vi "Get Language Name.vi"(8 "error in (no error)":errorcluster) -> (0 "error out":errorcluster, 1 "Path":map{string, path}(c390), 2 "Tag":string[](array[string]), 3 "Tag Name":string[](array[string]))   [LabVIEW 2025, in "Localization.lvlib"]
uses:
  Localization.lvlib
  <vilib>/Utility/config.llb/Read Key (String).vi
  Full User Interface/Full User Interface.lvlib
  <userlib>/_OpenG.lib/file/file.llb/openg_file.lvlib
  <vilib>/Utility/config.llb/NI_LVConfig.lvlib
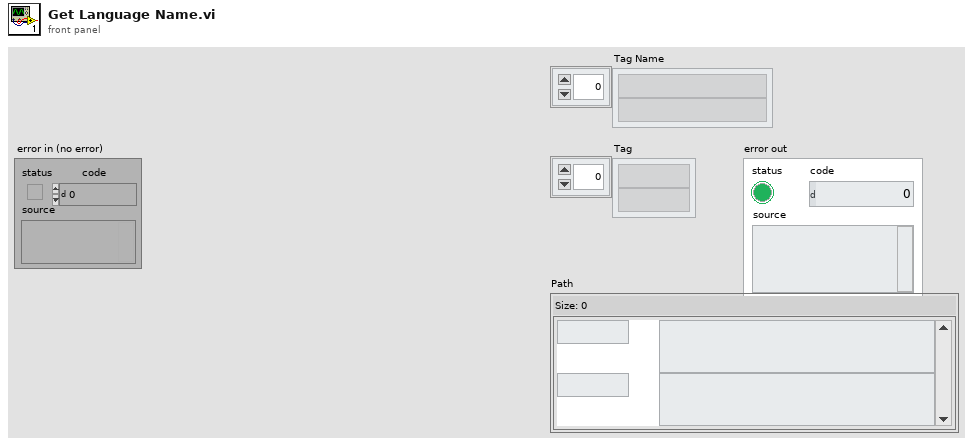
[diagram p1: front panel]
types:
  T1 = typedef "NI_LVConfig.lvlib/Config Data RefNum.ctl" = refnum<k1>
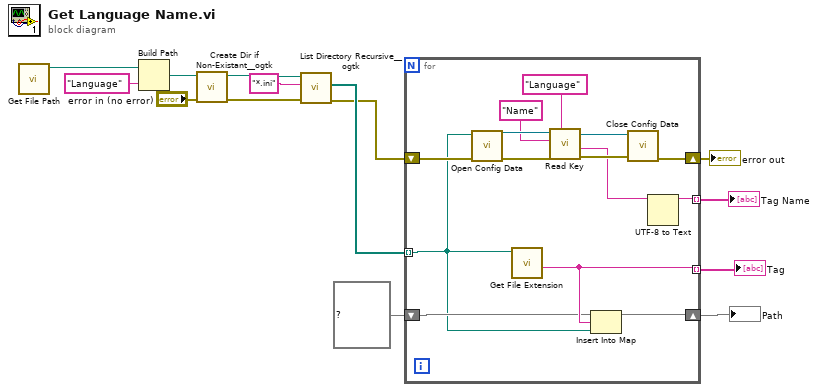
[diagram p0: block diagram]
diagram:
  n1 = call "Get File Path.vi"() -> ("Application Directory"=w14:path)  [unwired: 11 in]
  n2 = Build Path(base path=w14, name or relative path="Language") -> (appended path=w12:path)
  n3 = call <userlib>:"Create Dir if Non-Existant__ogtk.vi"("error in (no error)"="error in (no error)", "Directory Path"=w12) -> ("error out"=w7:errorcluster, "dup Directory Path"=w11:path)  [unwired: 7 in, 1 out]
  n4 = call <userlib>:"List Directory Recursive__ogtk.vi"("error in (no error)"=w7, "pattern"="*.ini", "Path"=w11) -> ("error out"=w6:errorcluster, "file paths"=w9:path[])  [unwired: 5 in, 2 out]
  n5 = for {
    tunnel: w9 -> [w15] mode=indexing
    tunnel: [w18] -> w8 mode=indexing
    shift-right: [w22] -> w4
    shift-left: w6 -> [w21]
    tunnel: [w19] -> w3 mode=indexing
    shift-right: [w16] -> w1
    shift-left: map{string, path} {} ("map") -> [w17]
    n6 = call <vilib>:"Open Config Data.vi"("error in (no error)"=w21, "configuration file path"=w15) -> ("error out"=w27:errorcluster, "refnum"=w28:T1)  [unwired: 7 in, 1 out]
    n7 = call <vilib>:"Get File Extension.vi"("file"=w15) -> ("filename without extension"=w18:string)  [unwired: 6 in, 4 out]
    n8 = call-poly <vilib>:"Read Key.vi"("section"="Language", "error in (no error)"=w27, "key"="Name", "refnum"=w28) -> ("error out"=w26:errorcluster, "value"=w20:string, "refnum out"=w25:T1)  [unwired: 4 in, 1 out]
    n9 = Insert Into Map(map in=w17, key=w18, value=w15) -> (map out=w16:map{string, path})  [unwired: 2 out]
    n10 = call <vilib>:"Close Config Data.vi"("error in (no error)"=w26, "refnum"=w25) -> ("error out"=w22:errorcluster)  [unwired: 8 in, 1 out]
    n11 = UTF-8 to Text(11:w20) -> (3:w19:string)  [unwired: 2 in, 1 out]
  }
  "Tag" <- w8
  "error out" <- w4
  "Tag Name" <- w3
  "Path" <- w1
